vi "Is Flat Type.vi"(8 "error in (no error)":errorcluster, 11 "LVArrayType in":refnum<class "LVArrayType.lvclass">) -> (0 "error out":errorcluster, 2 "Flat Type?":bool, 3 "LVArrayType out":refnum<class "LVArrayType.lvclass">)   [LabVIEW 2020, in "LVDataTypes.lvlib" / "LVArrayType.lvclass"]
uses:
  <vilib>/AppBuilder/Engine/WebServiceDescription/LVDataTypes/LVArrayType/LVArrayType.lvclass
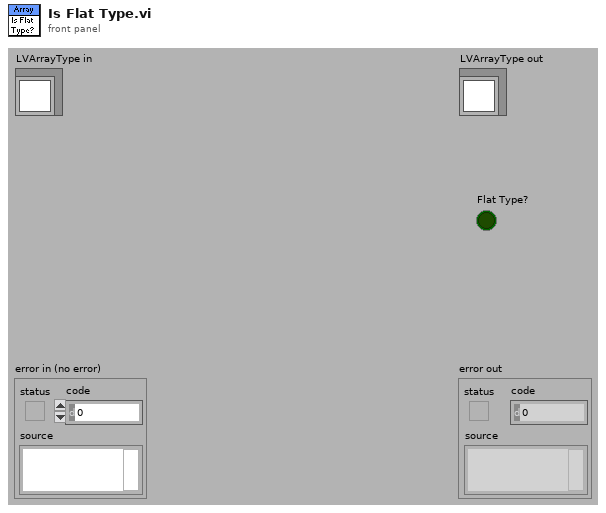
[diagram p1: front panel]
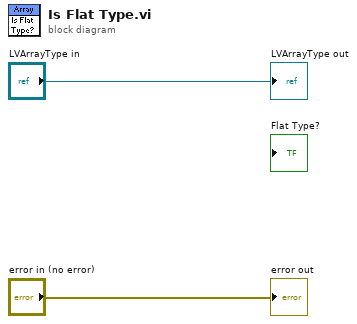
[diagram p0: block diagram]
diagram:
  "error out" <- "error in (no error)"
  "LVArrayType out" <- "LVArrayType in"
